vi "inpparam.vi"() -> (0 "1/m":dbl, 1 "b/Izz":dbl, 2 "lk/Iyy":dbl, 3 "lk/Ixx":dbl)   [LabVIEW 2015]
panel:
  in  "m":dbl=1.316
  in  "b":dbl=1.14e-07
  in  "Izz":dbl=3.57e-06
  in  "Iyy":dbl=3.57e-06
  in  "Ixx":dbl=3.57e-06
  in  "k":dbl=2.9814e-06
  in  "l":dbl=0.5
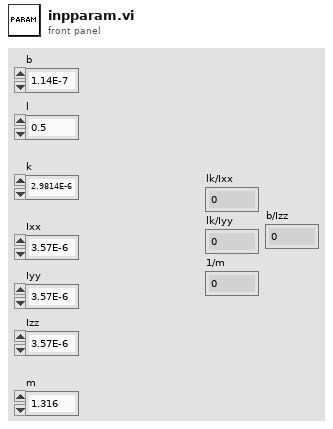
[diagram p1: front panel]
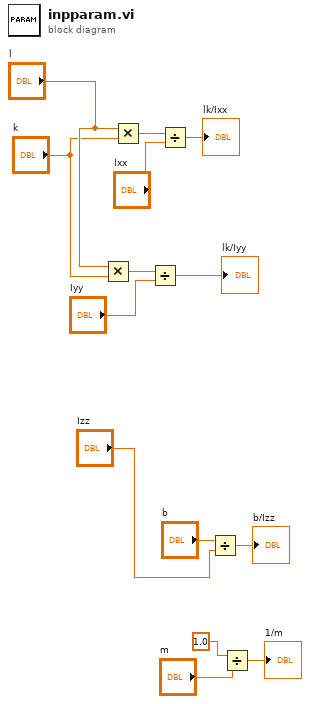
[diagram p0: block diagram]
diagram:
  n1 = Multiply(x="l", y="k") -> (x*y=w11:dbl)
  n2 = Multiply(x="l", y="k") -> (x*y=w14:dbl)
  n3 = Divide(x=w11, y="Iyy") -> (x/y=→"lk/Iyy":dbl)
  n4 = Divide(x=w14, y="Ixx") -> (x/y=→"lk/Ixx":dbl)
  n5 = Divide(x="b", y="Izz") -> (x/y=→"b/Izz":dbl)
  n6 = Divide(x=1.0, y="m") -> (x/y=→"1/m":dbl)
